vi "1D Inverse DST.vi"(11 "DST {X}":dbl[](array[numeric])) -> (0 "error":i32, 3 "X":dbl[](array[numeric]))   [LabVIEW 2024, in "NI_AALPro.lvlib"]
doc: "<p>Computes the inverse Discrete Sine Transform (DST) of the input sequence <strong>DST {X}</strong>. Wire data to the <strong>DST {X}</strong> input to determine the polymorphic instance to use or <a href=\"nihelplauncher://docs/csh?context=lvcore_lvhowto_selectingdefaultinstpolyvi\">manually select</a> the instance.\n</p>"
uses:
  NI_AALPro.lvlib
  <resource>/lvanlys.dll
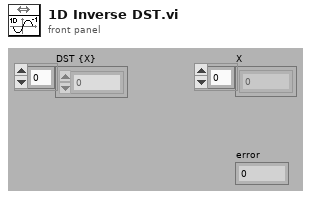
[diagram p1: front panel]
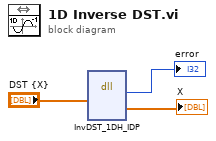
[diagram p0: block diagram]
diagram:
  n1 = dll-call lib="C:/Program Files (x86)/National Instruments/LabVIEW 2024/resource/lvanlys.*" fn="InvDST_1DH_IDP"("xH"="DST {X}") -> ("return type"=→"error":i32, "yH"=→"X":dbl[])  [unwired: 7 in, 2 out]
